vi "Autonomous.vi"   [LabVIEW 2017]
doc: "This VI starts when autonomous period begins, and will automatically be terminated when it ends. You can carry out timed or sensor driven operations directly to I/O or to subsystems without needing to return to the caller."
uses:
  <vilib>/Rock Robotics/WPI/Utilities/WPI_GetSetVariantRefNum.vi
  <vilib>/Rock Robotics/Network Tables/NT Read String.vi
types:
  T1 = typedef "WPI_JoystickDevRef.ctl" = cluster{"Device":T2}
  T2 = typedef "WPI_JoystickDeviceEnum.ctl" = enum16{"USB 0", "USB 1", "USB 2", "USB 3", "USB 4", "USB 5"}
  T3 = typedef "Command Status Info.ctl" = cluster{"Name":string, "Status":T4, "notifier out":T5}
  T4 = typedef "Completion Status.ctl" = enum16{"Successful", "Aborted", "Incomplete"}
  T5 = typedef "Completion Notifier.ctl" = refnum<notifier>
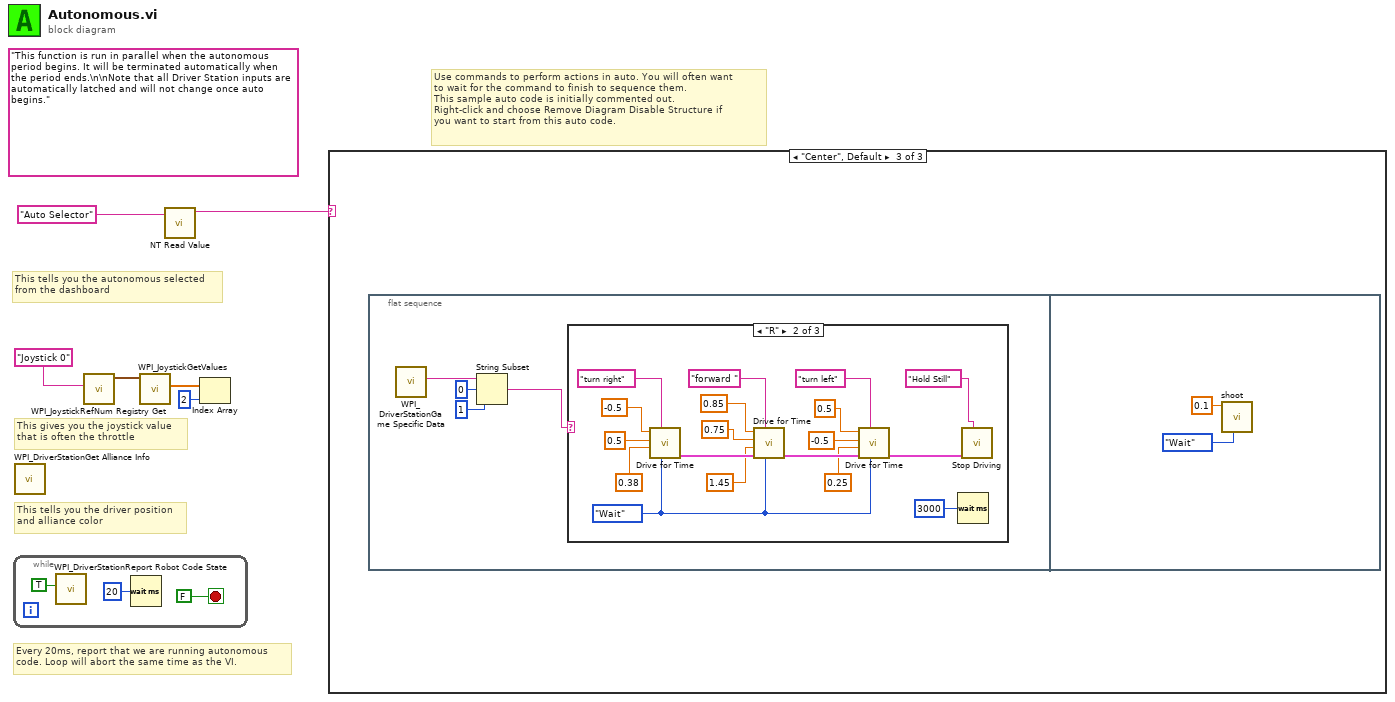
[diagram p0: block diagram]
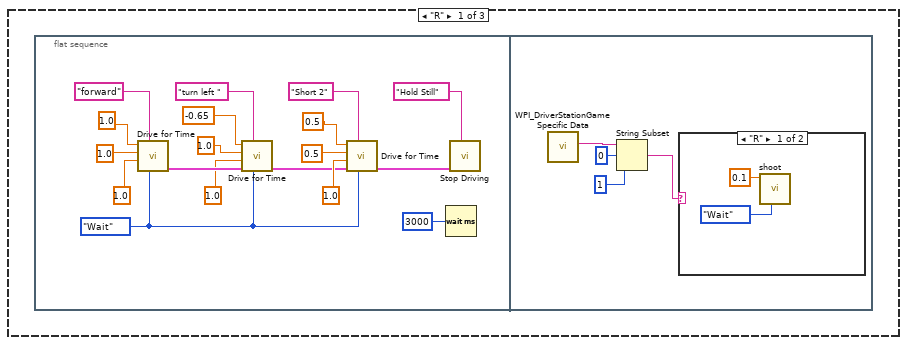
[diagram p2: hidden frame]
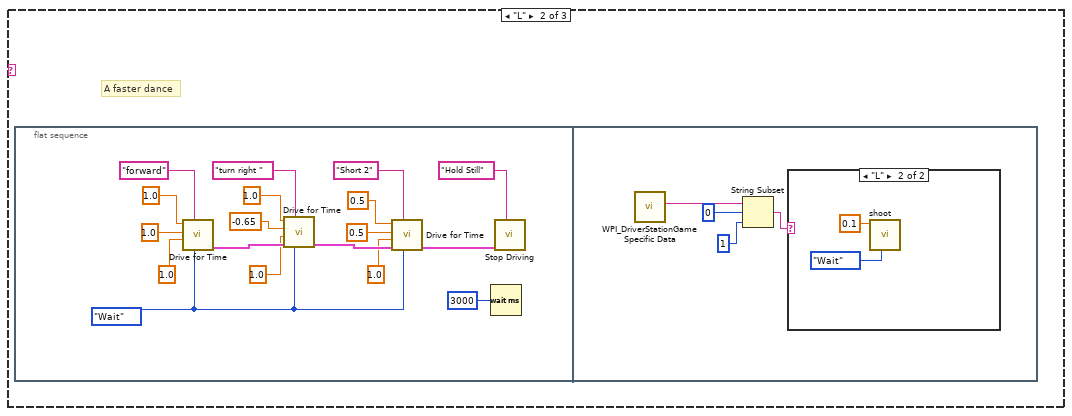
[diagram p4: hidden frame]
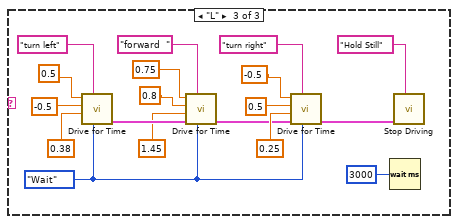
[diagram p7: hidden frame]
diagram:
  (unwired) "This function is run in parallel when the autonomous period begins. It will be terminated automatically when the period ends.\n\nNote that all Driver Station inputs are automatically latched and will not change once auto begins."
  # "This tells you the autonomous selected\nfrom the dashboard"
  # "Every 20ms, report that we are running autonomous\ncode. Loop will abort the same time as the VI."
  # "This gives you the joystick value\nthat is often the throttle"
  # "Use commands to perform actions in auto. You will often want\nto wait for the command to finish to sequence them.\nThis sample auto code is initially commented out. \nRight-click and choose Remove Diagram Disable Structure if\nyou want to start from this auto code."
  # "This tells you the driver position\nand alliance color"
  n1 = while {
    stop <- FALSE stop-if-true
    n2 = call <vilib>:"WPI_DriverStationReport Robot Code State.vi"("Autonomous"=TRUE) -> ()  [unwired: 10 in, 1 out]
    n3 = Wait (ms)(milliseconds to wait=u32 20) -> ()  [unwired: 1 out]
  }
  n4 = call <vilib>:"WPI_DriverStationGet Alliance Info.vi"() -> ()  [unwired: 12 out]
  n5 = call <vilib>:"WPI_JoystickRefNum Registry Get.vi"("refnum name"="Joystick 0") -> ("JoystickDevRef"=w5:T1)  [unwired: 1 in, 9 out]
  n6 = call <vilib>:"WPI_JoystickGetValues.vi"("JoystickDevRef"=w5) -> ("Axes"=w4:dbl[])  [unwired: 6 in, 4 out]
  n7 = call-poly <vilib>:"NT Read Value.vi"("Name"="Auto Selector") -> ("String"=w1:string)  [unwired: 9 in, 1 out]
  n8 = Index Array(array=w4, index=2) -> ()  [unwired: 1 out]
  n9 = case shown="\"Center\", Default" w1 {
    frame "R" {
      n10 = flat-sequence {
        frame #0 {
          w10 = enum16{"Start", "Wait"}."Wait" ("Synchronication")
          n11 = call "Drive for Time.vi"("Synchronization"=w10, "Description"="forward", "Seconds"=1.0 ("Delay (s)"), "Right Speed"=1.0 ("X axis value"), "Left Speed"=1.0 ("X axis value")) -> ("Command Info Out"=w27:T3)  [unwired: 5 in, 1 out]
          n12 = call "Drive for Time.vi"("Synchronization"=w10, "Description"="turn left ", "Command Info In"=w27, "Seconds"=1.0 ("Delay (s)"), "Right Speed"=1.0 ("X axis value"), "Left Speed"=-0.65 ("X axis value")) -> ("Command Info Out"=w12:T3)  [unwired: 4 in, 1 out]
          n13 = call "Drive for Time.vi"("Synchronization"=w10, "Description"="Short 2", "Command Info In"=w12, "Seconds"=1.0 ("Delay (s)"), "Right Speed"=0.5 ("X axis value"), "Left Speed"=0.5 ("X axis value")) -> ("Command Info Out"=w11:T3)  [unwired: 4 in, 1 out]
          n14 = Wait (ms)(milliseconds to wait=u32 3000 ("millisecond timer value")) -> ()  [unwired: 1 out]
          n15 = call "Stop Driving.vi"("Description"="Hold Still", "Command Info In"=w11) -> ()  [unwired: 9 in, 1 out]
        }
        frame #1 {
          n16 = call <vilib>:"WPI_DriverStationGame Specific Data.vi"() -> ("Game Specific Data"=w31:string)  [unwired: 11 in]
          n17 = String Subset(string=w31, offset (0)=0, length (rest)=1 ("length (rest)")) -> (substring=w28:string)
          n18 = case shown="\"R\"" w28 {
            frame "R" {
              n19 = call "shoot.vi"("Synchronization"=enum16{"Start", "Wait"}."Wait", "shooterSetpoint"=0.1) -> ()  [unwired: 9 in, 1 out]
            }
            frame "L", Default {
            }
          }
        }
      }
    }
    frame "L" {
      # "A faster dance"
      n20 = flat-sequence {
        frame #0 {
          w34 = enum16{"Start", "Wait"}."Wait" ("Synchronication")
          n21 = call "Drive for Time.vi"("Synchronization"=w34, "Description"="forward", "Seconds"=1.0 ("Delay (s)"), "Right Speed"=1.0 ("X axis value"), "Left Speed"=1.0 ("X axis value")) -> ("Command Info Out"=w49:T3)  [unwired: 5 in, 1 out]
          n22 = call "Drive for Time.vi"("Synchronization"=w34, "Description"="turn right ", "Command Info In"=w49, "Seconds"=1.0 ("Delay (s)"), "Right Speed"=-0.65 ("X axis value"), "Left Speed"=1.0 ("X axis value")) -> ("Command Info Out"=w50:T3)  [unwired: 4 in, 1 out]
          n23 = call "Drive for Time.vi"("Synchronization"=w34, "Description"="Short 2", "Command Info In"=w50, "Seconds"=1.0 ("Delay (s)"), "Right Speed"=0.5 ("X axis value"), "Left Speed"=0.5 ("X axis value")) -> ("Command Info Out"=w51:T3)  [unwired: 4 in, 1 out]
          n24 = Wait (ms)(milliseconds to wait=u32 3000 ("millisecond timer value")) -> ()  [unwired: 1 out]
          n25 = call "Stop Driving.vi"("Description"="Hold Still", "Command Info In"=w51) -> ()  [unwired: 9 in, 1 out]
        }
        frame #1 {
          n26 = call <vilib>:"WPI_DriverStationGame Specific Data.vi"() -> ("Game Specific Data"=w55:string)  [unwired: 11 in]
          n27 = String Subset(string=w55, offset (0)=0, length (rest)=1 ("length (rest)")) -> (substring=w52:string)
          n28 = case shown="\"L\"" w52 {
            frame "R", Default {
            }
            frame "L" {
              n29 = call "shoot.vi"("Synchronization"=enum16{"Start", "Wait"}."Wait", "shooterSetpoint"=0.1) -> ()  [unwired: 9 in, 1 out]
            }
          }
        }
      }
    }
    frame "Center", Default {
      n30 = flat-sequence {
        frame #0 {
          n31 = call <vilib>:"WPI_DriverStationGame Specific Data.vi"() -> ("Game Specific Data"=w61:string)  [unwired: 11 in]
          n32 = String Subset(string=w61, offset (0)=0, length (rest)=1 ("length (rest)")) -> (substring=w58:string)
          n33 = case shown="\"R\"" w58 {
            frame Default {
            }
            frame "R" {
              w76 = enum16{"Start", "Wait"}."Wait" ("Synchronication")
              n34 = call "Drive for Time.vi"("Synchronization"=w76, "Description"="turn right", "Seconds"=0.38 ("Delay (s)"), "Right Speed"=0.5 ("X axis value"), "Left Speed"=-0.5 ("X axis value")) -> ("Command Info Out"=w77:T3)  [unwired: 5 in, 1 out]
              n35 = call "Drive for Time.vi"("Synchronization"=w76, "Description"="forward ", "Command Info In"=w77, "Seconds"=1.45 ("Delay (s)"), "Right Speed"=0.75 ("X axis value"), "Left Speed"=0.85 ("X axis value")) -> ("Command Info Out"=w78:T3)  [unwired: 4 in, 1 out]
              n36 = call "Drive for Time.vi"("Synchronization"=w76, "Description"="turn left", "Command Info In"=w78, "Seconds"=0.25 ("Delay (s)"), "Right Speed"=-0.5 ("X axis value"), "Left Speed"=0.5 ("X axis value")) -> ("Command Info Out"=w79:T3)  [unwired: 4 in, 1 out]
              n37 = Wait (ms)(milliseconds to wait=u32 3000 ("millisecond timer value")) -> ()  [unwired: 1 out]
              n38 = call "Stop Driving.vi"("Description"="Hold Still", "Command Info In"=w79) -> ()  [unwired: 9 in, 1 out]
            }
            frame "L" {
              w80 = enum16{"Start", "Wait"}."Wait" ("Synchronication")
              n39 = call "Drive for Time.vi"("Synchronization"=w80, "Description"="turn left", "Seconds"=0.38 ("Delay (s)"), "Right Speed"=-0.5 ("X axis value"), "Left Speed"=0.5 ("X axis value")) -> ("Command Info Out"=w97:T3)  [unwired: 5 in, 1 out]
              n40 = call "Drive for Time.vi"("Synchronization"=w80, "Description"="forward  ", "Command Info In"=w97, "Seconds"=1.45 ("Delay (s)"), "Right Speed"=0.8 ("X axis value"), "Left Speed"=0.75 ("X axis value")) -> ("Command Info Out"=w82:T3)  [unwired: 4 in, 1 out]
              n41 = call "Drive for Time.vi"("Synchronization"=w80, "Description"="turn right", "Command Info In"=w82, "Seconds"=0.25 ("Delay (s)"), "Right Speed"=0.5 ("X axis value"), "Left Speed"=-0.5 ("X axis value")) -> ("Command Info Out"=w81:T3)  [unwired: 4 in, 1 out]
              n42 = Wait (ms)(milliseconds to wait=u32 3000 ("millisecond timer value")) -> ()  [unwired: 1 out]
              n43 = call "Stop Driving.vi"("Description"="Hold Still", "Command Info In"=w81) -> ()  [unwired: 9 in, 1 out]
            }
          }
        }
        frame #1 {
          n44 = call "shoot.vi"("Synchronization"=enum16{"Start", "Wait"}."Wait", "shooterSetpoint"=0.1) -> ()  [unwired: 9 in, 1 out]
        }
      }
    }
  }
